vi "Upgraded_Live_Version.vi"() -> ()   [LabVIEW 2023]
panel:
  in  "Get ROI":bool
  in  "Height":u16
  in  "Y":u16
  in  "Width":u16
  in  "X":u16
  out "Trigger Mode":i32
  in  "Trigger In Behaviour":string(combo)
  out "Exp. out":i32
  in  "Trigger Out Behaviour":string(combo)
  out "Boolean":bool
  in  "Scan Direction Reset":bool
  out "Scan Line Time":dbl format="%#_14g"
  in  "Scan Width":dbl
  in  "Scan Line Delay":dbl
  in  "Scan Direction":string(combo)
  in  "Scan Mode":string(combo)
  in  "Exposure Time":dbl
  in  "Live":bool
  in  "Camera Status":bool
  in  "Uninit":bool
  in  "Live stop":bool
  in  "Live start":bool
  in  "Open":bool
  # "SimpleLiveAppProgrammableScanMode.vi\n\nDescription:\nThis sample code lets the user use programmable scan\n mode in an event driven structure.\n\nSteps to run:\n1. Click \"Run\"\n2. Click \"Open\"\n3. Enter Exposure Time\n4. Select Scan Mode. \n5. Set Scan Line Delay or Scan Width\n6. Select Scan Direction\n7. Click \"Live start\"\n8. Click \"Live stop\"\n9. Click \"Close\""
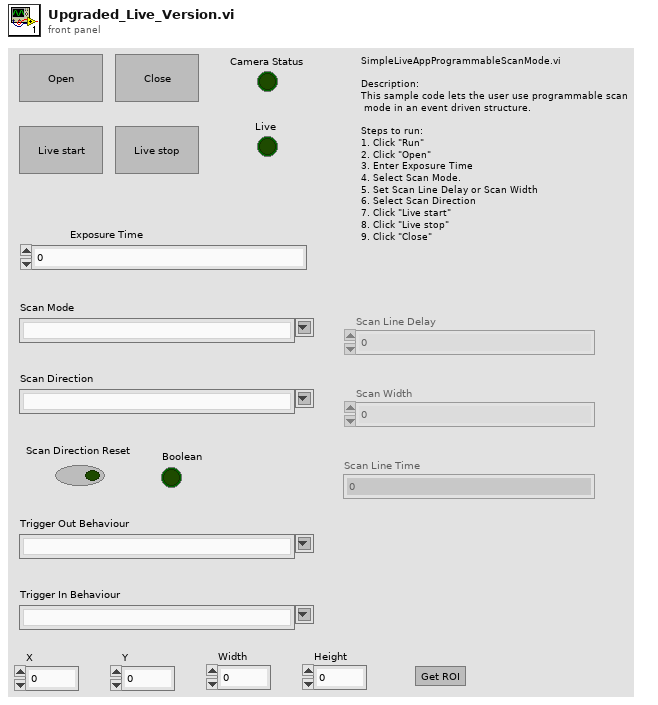
[diagram p1: front panel]
types:
  T1 = enum8{"Enabled", "Disabled", "Disabled and Grayed Out"}
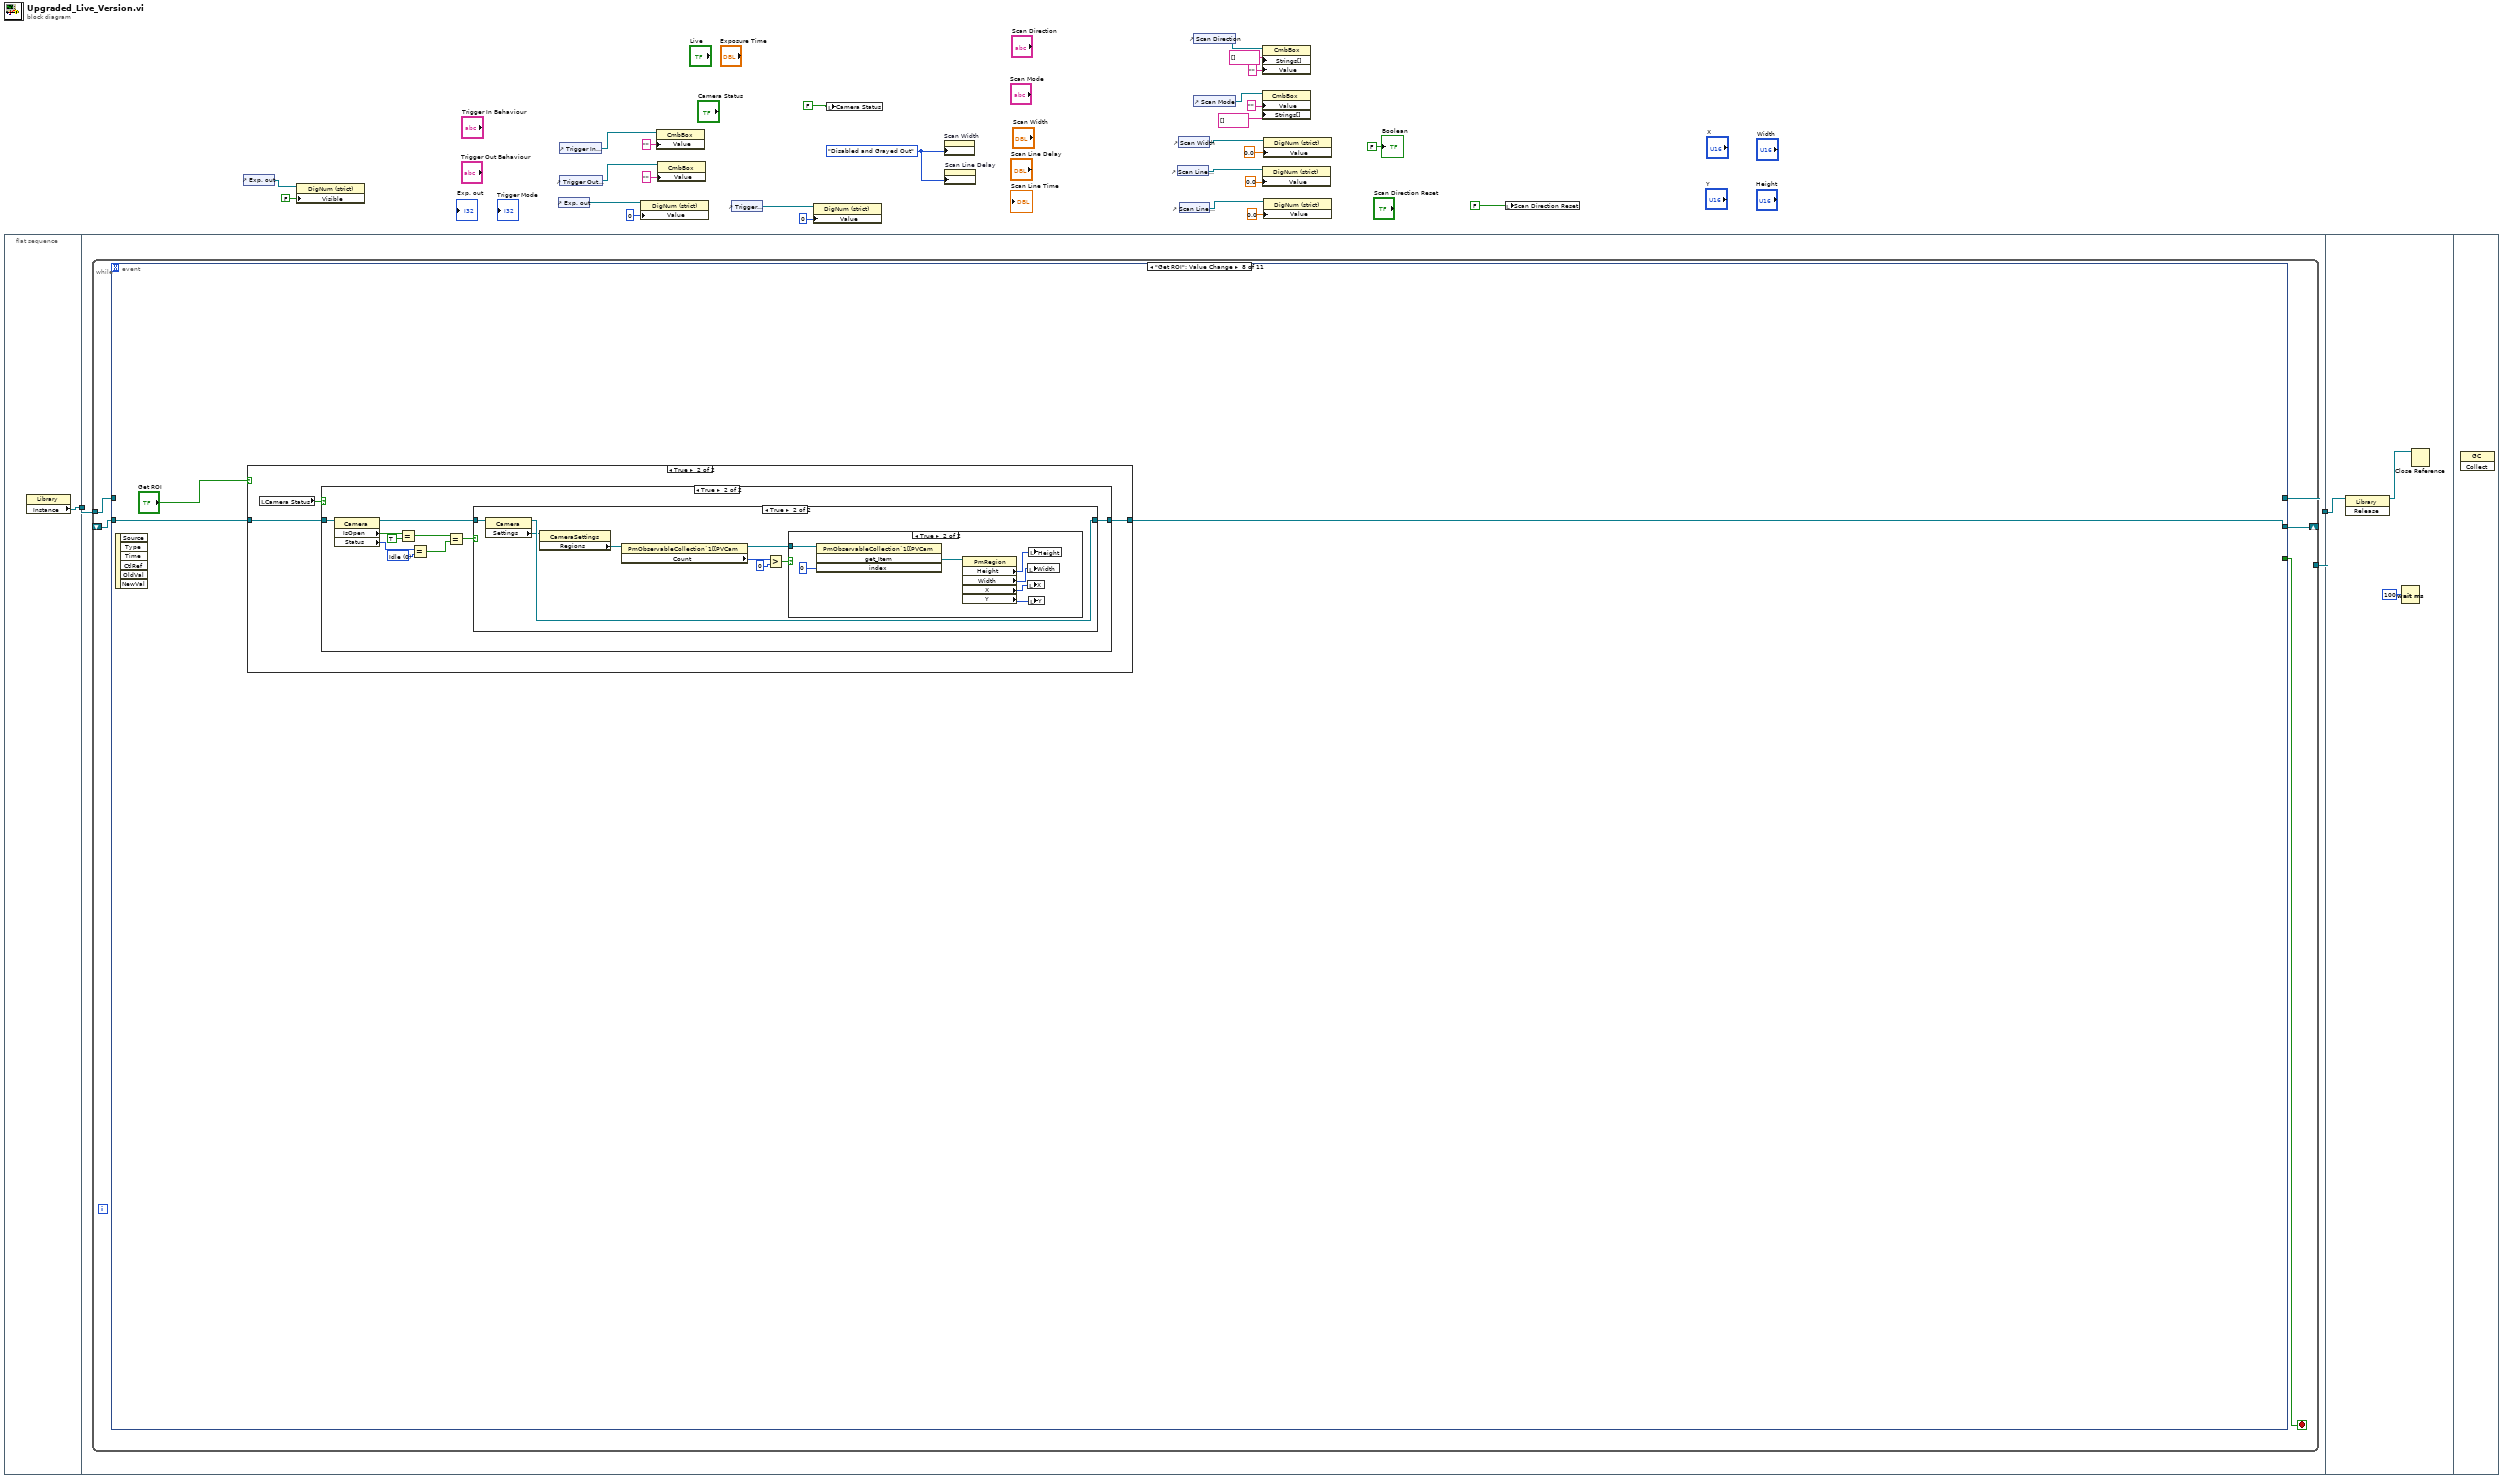
[diagram p0: block diagram]
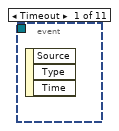
[diagram p2: hidden frame]
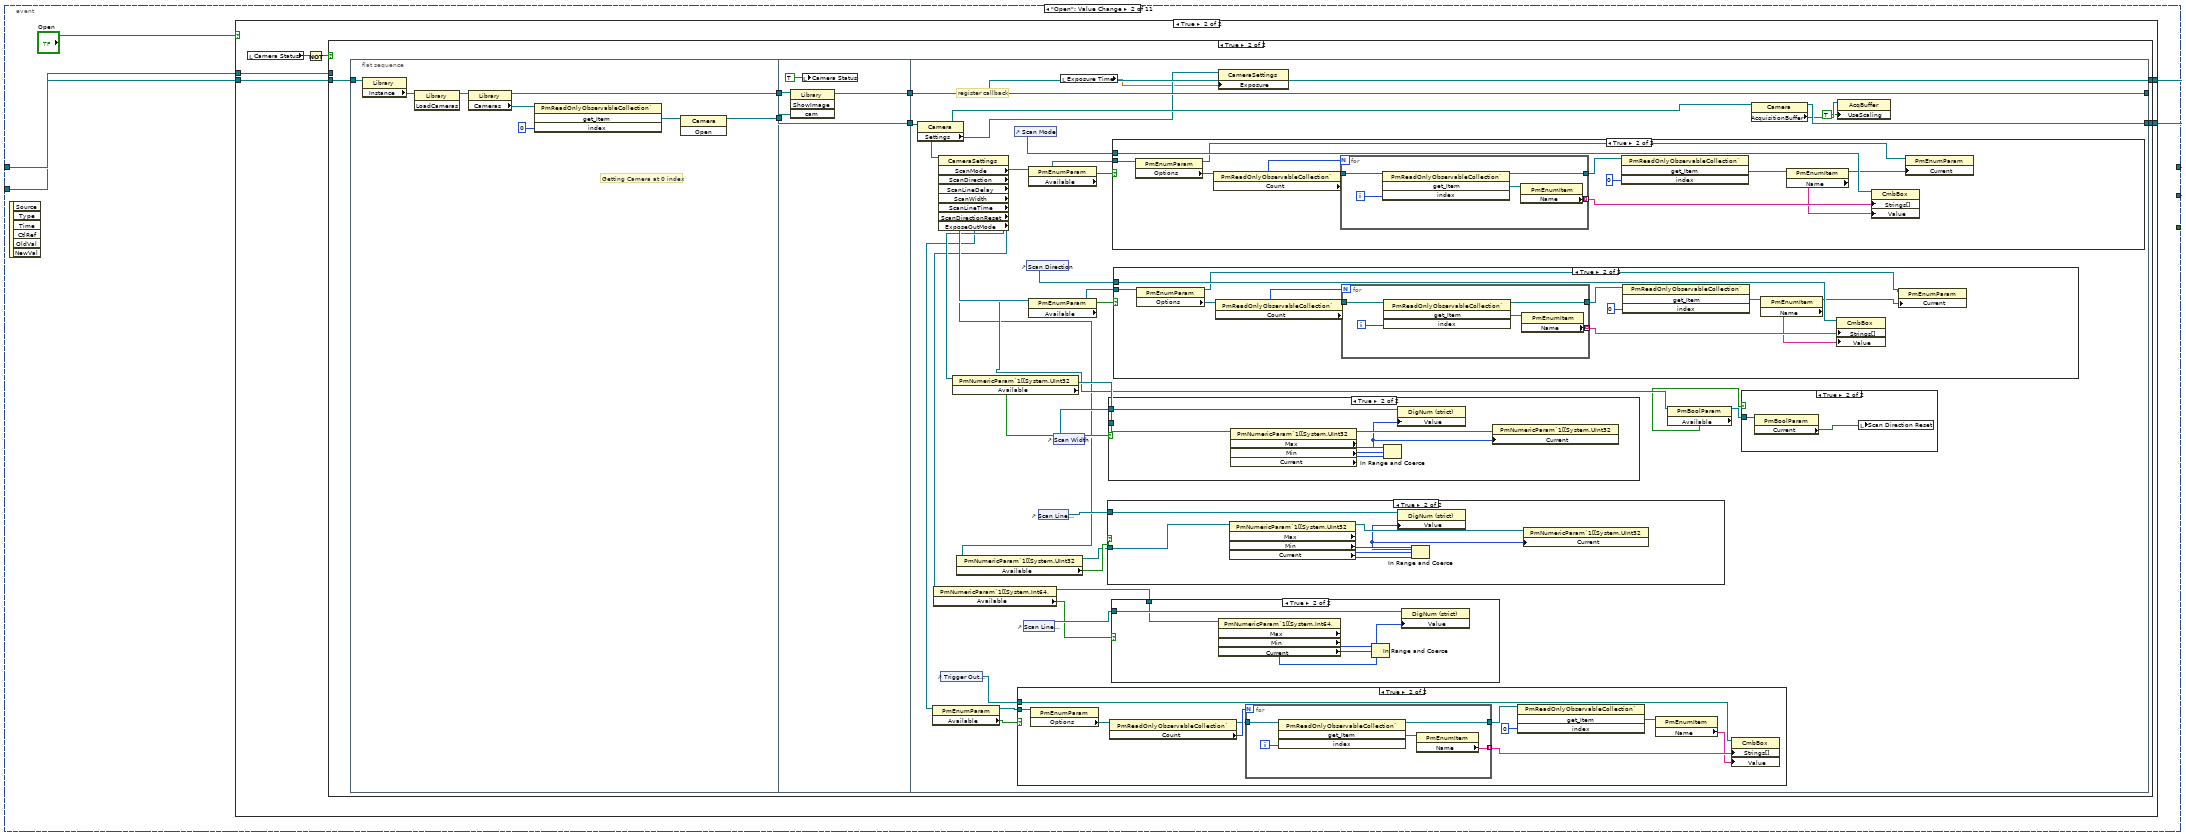
[diagram p3: hidden frame]
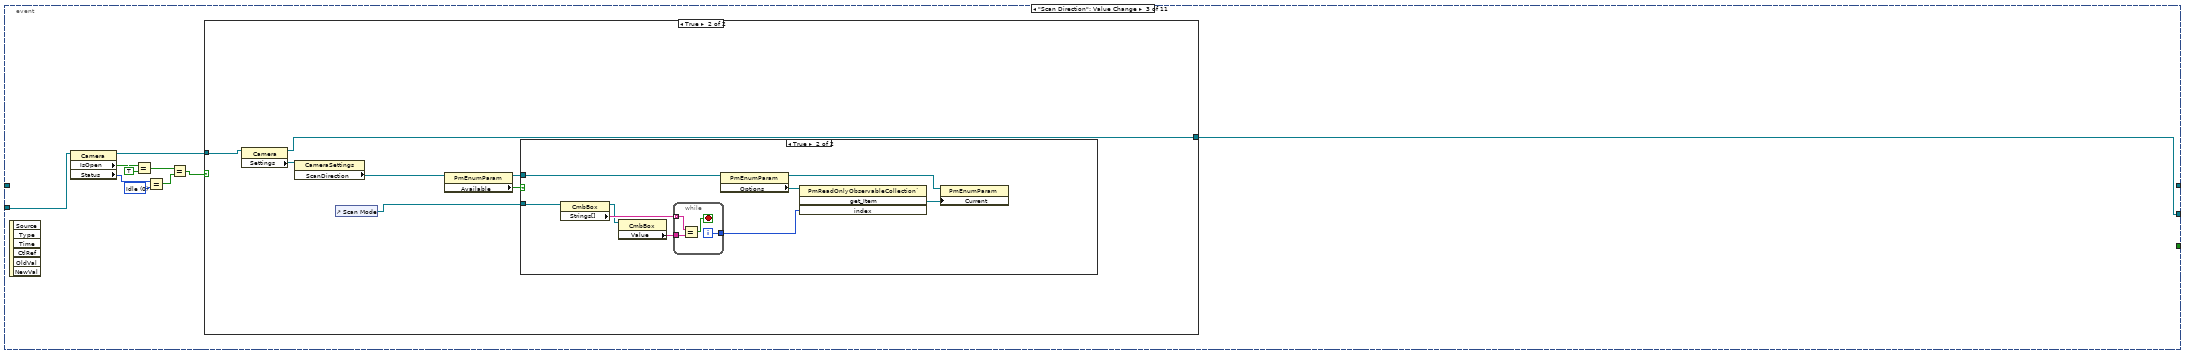
[diagram p13: hidden frame]
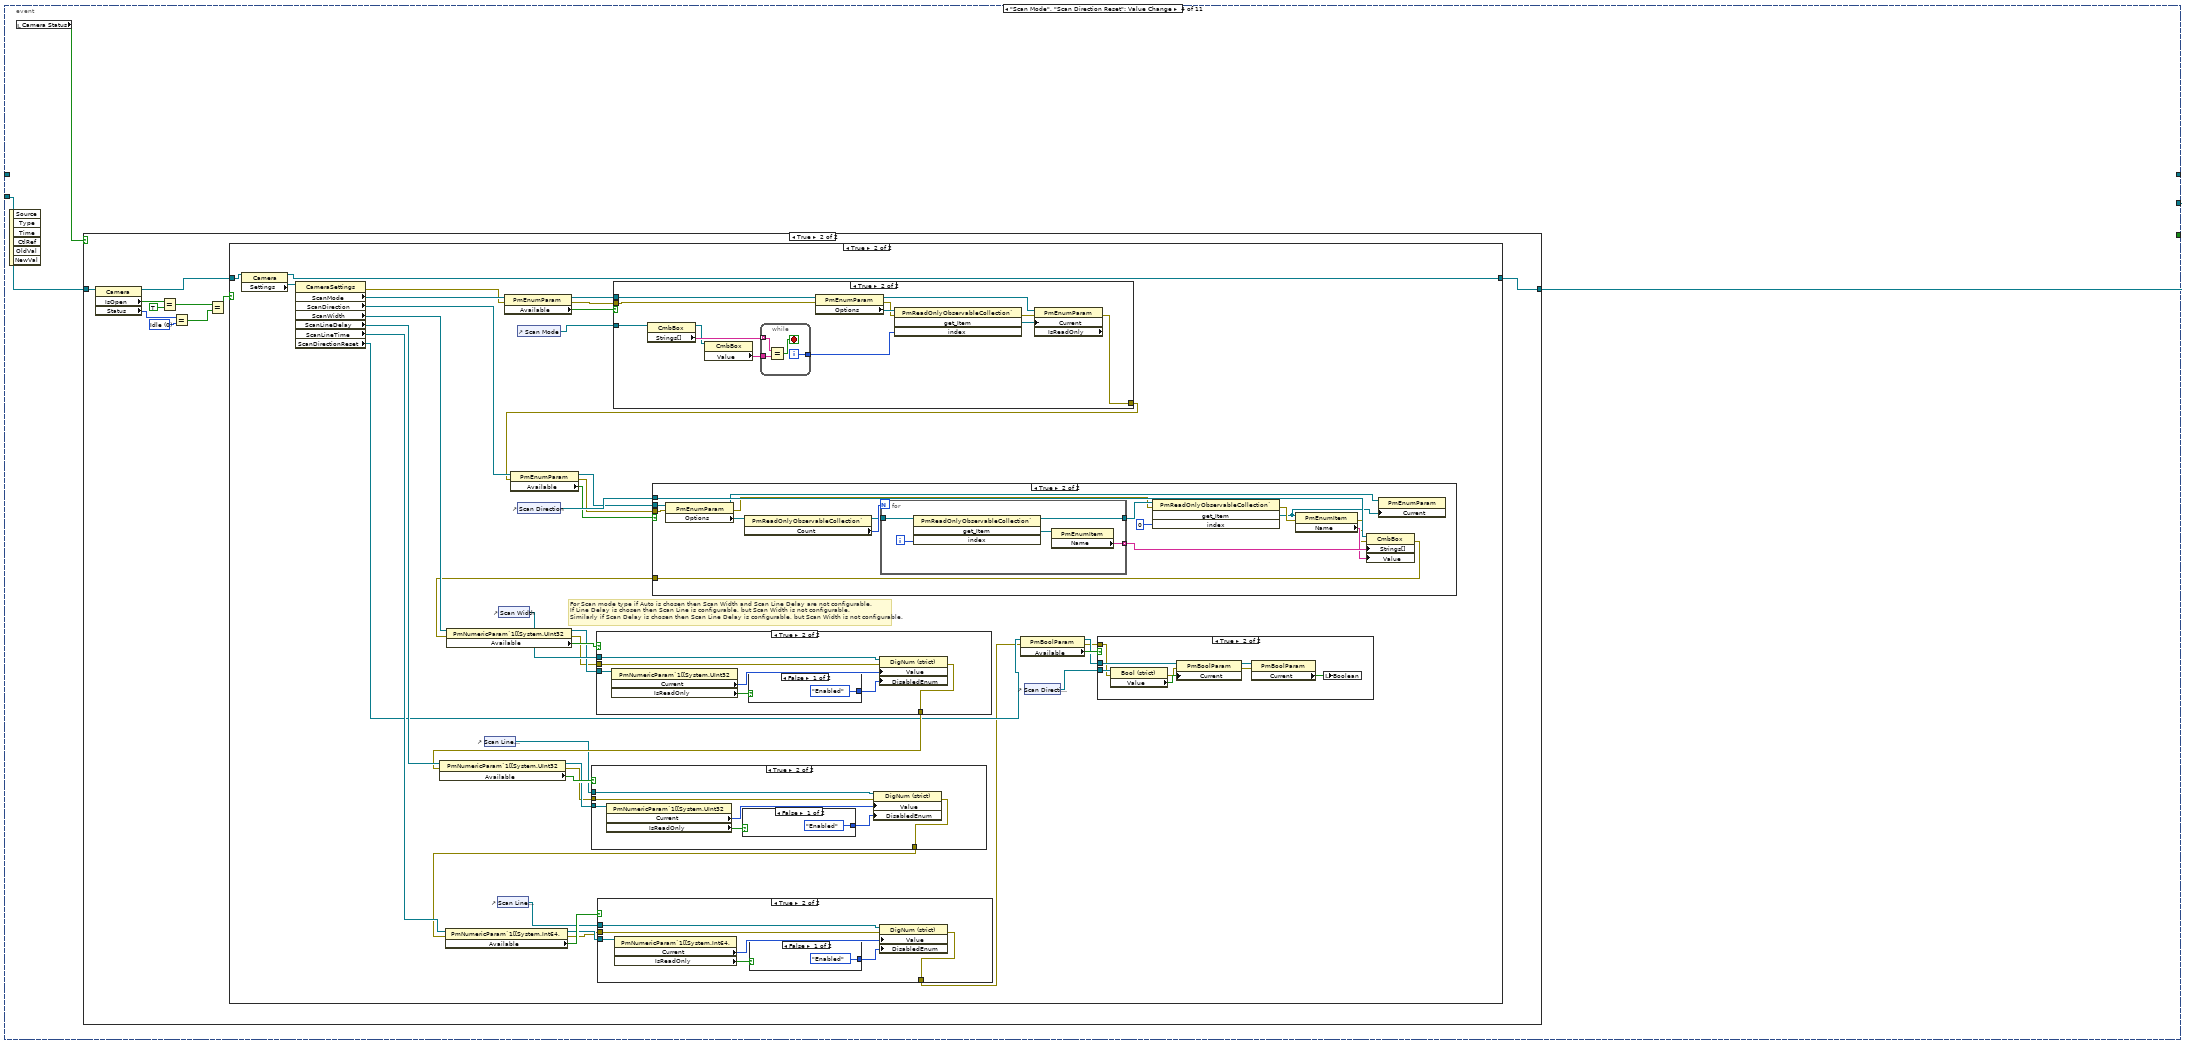
[diagram p16: hidden frame]
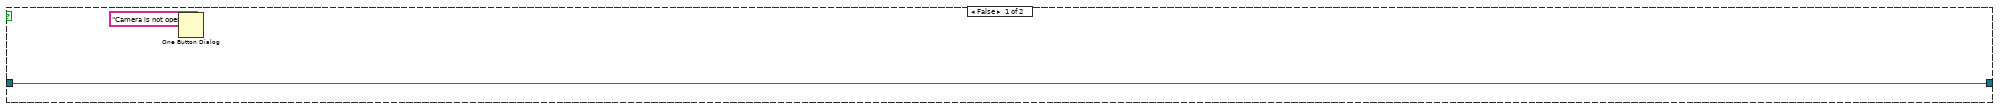
[diagram p17: hidden frame]
diagram:
  w13 = T1."Disabled and Grayed Out" ("Disabled")
  n1 = flat-sequence {
    tunnel: [w29] -> w28
    tunnel: w28 -> [w31]
    tunnel: [w30] -> w27
    tunnel: w27 -> [w652]
    frame #0 {
      n2 = property class="Library"() -> ("Instance"=w29:refnum<k24>)  [unwired: 2 in, 2 out]
    }
    frame #1 {
      n3 = while {
        tunnel: w31 -> [w36]
        shift-right: [w35] -> _
        shift-left: _ -> [w33]
        tunnel: [w34] -> w30
        stop <- w32 stop-if-true
        n4 = event shown="[7] \"Get ROI\": Value Change" {
          selector: _ -> [_ _ _ _ _ _ _ _ _ _ _]
          dyn-events: _ -> [_ _ _ _ _ _ _ _ _ _ _]
          timeout: _ -> [_ _ _ _ _ _ _ _ _ _ _]
          tunnel: w36 -> [_ w41 _ _ _ _ w464 _ w569 _ w624]
          tunnel: [_ w40 w177 w209 w341 w405 w465 w532 w570 w599 w625] -> w35
          tunnel: [_ w39 _ _ _ _ w464 _ w569 _ w624] -> w34
          tunnel: w33 -> [_ w38 w181 w210 w347 w407 w466 w533 w571 w600 w626]
          tunnel: [_ _ _ _ _ _ _ _ _ _ w623] -> w32
          event Timeout {
            n5 = event-data() -> ()  [unwired: 1 in, 3 out]
          }
          event "Open": Value Change {
            n6 = event-data() -> ()  [unwired: 1 in, 6 out]
            n7 = case shown="True" "Open" {
              tunnel: w41 -> [w43 w49]
              tunnel: [w42 w48] -> w40
              tunnel: [w43 w47] -> w39
              tunnel: w38 -> [w42 w44]
              frame False {
              }
              frame True {
                n8 = local read "Camera Status"() -> (w46:bool)
                n9 = Not(x=w46) -> (.not. x?=w45:bool)
                n10 = case shown="True" w45 {
                  tunnel: w49 -> [w50 w56]
                  tunnel: [w51 w55] -> w48
                  tunnel: [w50 w54] -> w47
                  tunnel: w44 -> [w51 _]
                  frame False {
                  }
                  frame True {
                    n11 = flat-sequence {
                      tunnel: w56 -> [w61]
                      tunnel: [w63] -> w58
                      tunnel: [w62] -> w57
                      tunnel: w58 -> [w69]
                      tunnel: w57 -> [w70]
                      tunnel: [w70] -> w53
                      tunnel: [w68] -> w52
                      tunnel: [w105] -> w54
                      tunnel: [w85] -> w55
                      tunnel: w53 -> [w104]
                      tunnel: w52 -> [w105]
                      frame #0 {
                        # "Getting Camera at 0 index"
                        n12 = property class="Library"(reference=w61) -> ("Instance"=w60:refnum<k24>)  [unwired: 1 in, 2 out]
                        n13 = invoke class="Library" method="LoadCameras"(reference=w60) -> (reference out=w59:refnum<k24>)  [unwired: 2 in, 2 out]
                        n14 = property class="Library"(reference=w59) -> (reference out=w63:refnum<k24>, "Cameras"=w66:refnum<k24>)  [unwired: 1 in, 1 out]
                        n15 = invoke class="PmReadOnlyObservableCollection`" method="get_Item"(reference=w66, "index"=0) -> ("get_Item"=w64:refnum<k24>)  [unwired: 2 in, 3 out]
                        n16 = invoke class="Camera" method="Open"(reference=w64) -> (reference out=w62:refnum<k24>)  [unwired: 2 in, 2 out]
                      }
                      frame #1 {
                        n17 = invoke class="Library" method="ShowImage"(reference=w69, "cam"=w70) -> (reference out=w68:refnum<k24>)  [unwired: 2 in, 3 out]
                        n18 = local write "Camera Status"(TRUE ("Camera Status")) -> ()
                      }
                      frame #2 {
                        # "register callback"
                        n19 = property class="Camera"(reference=w104) -> (reference out=w86:refnum<k24>, "Settings"=w75:refnum<k24>)  [unwired: 1 in, 1 out]
                        n20 = property class="CameraSettings"(reference=w75) -> ("ScanMode"=w103:refnum<k24>, "ScanDirection"=w99:refnum<k24>, "ScanLineDelay"=w94:refnum<k24>, "ScanWidth"=w81:refnum<k24>, "ScanLineTime"=w73:refnum<k24>, "ScanDirectionReset"=w89:refnum<k24>, "ExposeOutMode"=w77:refnum<k24>)  [unwired: 1 in, 2 out]
                        n21 = property class="PmEnumParam"(reference=w77) -> (reference out=w78:refnum<k24>, "Available"=w79:bool)  [unwired: 1 in, 1 out]
                        n22 = property class="PmNumericParam`1[[System.Int64,"(reference=w73) -> (reference out=w71:refnum<k24>, "Available"=w72:bool)  [unwired: 1 in, 1 out]
                        n23 = control-ref of="Trigger Out Behaviour"() -> (w76:refnum<vi>)
                        n24 = property class="PmNumericParam`1[[System.UInt32"(reference=w94) -> (reference out=w92:refnum<k24>, "Available"=w93:bool)  [unwired: 1 in, 1 out]
                        n25 = property class="PmNumericParam`1[[System.UInt32"(reference=w81) -> (reference out=w80:refnum<k24>, "Available"=w82:bool)  [unwired: 1 in, 1 out]
                        n26 = control-ref of="Scan Mode"() -> (w100:refnum<vi>)
                        n27 = case shown="True" w79 {
                          tunnel: w78 -> [_ w115]
                          tunnel: w76 -> [_ w106]
                          frame False {
                          }
                          frame True {
                            n28 = property class="PmEnumParam"(reference=w115) -> ("Options"=w114:refnum<k24>)  [unwired: 1 in, 2 out]
                            n29 = property class="PmReadOnlyObservableCollection`"(reference=w114) -> (reference out=w112:refnum<k24>, "Count"=w113:i32)  [unwired: 1 in, 1 out]
                            n30 = for {
                              N: w113 -> [_]
                              tunnel: w112 -> [w120]
                              tunnel: [w117] -> w109
                              tunnel: [w116] -> w108 mode=indexing
                              i -> [w119]
                              n31 = invoke class="PmReadOnlyObservableCollection`" method="get_Item"(reference=w120, "index"=w119) -> (reference out=w117:refnum<k24>, "get_Item"=w118:refnum<k24>)  [unwired: 2 in, 2 out]
                              n32 = property class="PmEnumItem"(reference=w118) -> ("Name"=w116:string)  [unwired: 1 in, 2 out]
                            }
                            n33 = invoke class="PmReadOnlyObservableCollection`" method="get_Item"(reference=w109, "index"=0) -> ("get_Item"=w110:refnum<k24>)  [unwired: 2 in, 3 out]
                            n34 = property class="PmEnumItem"(reference=w110) -> ("Name"=w107:string)  [unwired: 1 in, 2 out]
                            n35 = property class="CmbBox"(reference=w106, "Strings[]"=w108, "Value"=w107) -> ()  [unwired: 1 in, 2 out]
                          }
                        }
                        n36 = control-ref of="Scan Line Time"() -> (w90:refnum<vi>)
                        n37 = control-ref of="Scan Direction"() -> (w96:refnum<vi>)
                        n38 = property class="PmEnumParam"(reference=w103) -> (reference out=w101:refnum<k24>, "Available"=w102:bool)  [unwired: 1 in, 1 out]
                        n39 = property class="PmEnumParam"(reference=w99) -> (reference out=w97:refnum<k24>, "Available"=w98:bool)  [unwired: 1 in, 1 out]
                        n40 = control-ref of="Scan Line Delay"() -> (w91:refnum<vi>)
                        n41 = control-ref of="Scan Width"() -> (w95:refnum<vi>)
                        n42 = local read "Exposure Time"() -> (w74:dbl)
                        n43 = case shown="True" w82 {
                          tunnel: w91 -> [_ w132]
                          tunnel: w80 -> [_ w131]
                          frame False {
                          }
                          frame True {
                            n44 = property class="PmNumericParam`1[[System.UInt32"(reference=w131) -> (reference out=w130:refnum<k24>, "Max"=w133:u32, "Min"=w134:u32, "Current"=w135:u32)  [unwired: 1 in, 1 out]
                            n45 = In Range and Coerce(upper limit=w133, x=w135, lower limit=w134) -> (coerced(x)=w129:u32)  [unwired: 1 out]
                            n46 = property class="DigNum (strict)"(reference=w132, "Value"=w129) -> ()  [unwired: 1 in, 2 out]
                            n47 = property class="PmNumericParam`1[[System.UInt32"(reference=w130, "Current"=w129) -> ()  [unwired: 1 in, 2 out]
                          }
                        }
                        n48 = case shown="True" w93 {
                          tunnel: w95 -> [_ w139]
                          tunnel: w92 -> [_ w138]
                          frame False {
                          }
                          frame True {
                            n49 = property class="PmNumericParam`1[[System.UInt32"(reference=w138) -> (reference out=w137:refnum<k24>, "Max"=w140:u32, "Min"=w141:u32, "Current"=w142:u32)  [unwired: 1 in, 1 out]
                            n50 = In Range and Coerce(upper limit=w140, x=w142, lower limit=w141) -> (coerced(x)=w136:u32)  [unwired: 1 out]
                            n51 = property class="DigNum (strict)"(reference=w139, "Value"=w136) -> ()  [unwired: 1 in, 2 out]
                            n52 = property class="PmNumericParam`1[[System.UInt32"(reference=w137, "Current"=w136) -> ()  [unwired: 1 in, 2 out]
                          }
                        }
                        n53 = case shown="True" w72 {
                          tunnel: w90 -> [_ w124]
                          tunnel: w71 -> [_ w123]
                          frame False {
                          }
                          frame True {
                            n54 = property class="PmNumericParam`1[[System.Int64,"(reference=w123) -> ("Max"=w125:i64, "Min"=w126:i64, "Current"=w127:i64)  [unwired: 1 in, 2 out]
                            n55 = In Range and Coerce(upper limit=w125, x=w127, lower limit=w126) -> (coerced(x)=w128:i64)  [unwired: 1 out]
                            n56 = property class="DigNum (strict)"(reference=w124, "Value"=w128) -> ()  [unwired: 1 in, 2 out]
                          }
                        }
                        n57 = case shown="True" w102 {
                          tunnel: w101 -> [_ w171]
                          tunnel: w100 -> [_ w163]
                          frame False {
                          }
                          frame True {
                            n58 = property class="PmEnumParam"(reference=w171) -> (reference out=w162:refnum<k24>, "Options"=w170:refnum<k24>)  [unwired: 1 in, 1 out]
                            n59 = property class="PmReadOnlyObservableCollection`"(reference=w170) -> (reference out=w168:refnum<k24>, "Count"=w169:i32)  [unwired: 1 in, 1 out]
                            n60 = for {
                              N: w169 -> [_]
                              tunnel: w168 -> [w176]
                              tunnel: [w173] -> w166
                              tunnel: [w172] -> w165 mode=indexing
                              i -> [w175]
                              n61 = invoke class="PmReadOnlyObservableCollection`" method="get_Item"(reference=w176, "index"=w175) -> (reference out=w173:refnum<k24>, "get_Item"=w174:refnum<k24>)  [unwired: 2 in, 2 out]
                              n62 = property class="PmEnumItem"(reference=w174) -> ("Name"=w172:string)  [unwired: 1 in, 2 out]
                            }
                            n63 = invoke class="PmReadOnlyObservableCollection`" method="get_Item"(reference=w166, "index"=0) -> ("get_Item"=w161:refnum<k24>)  [unwired: 2 in, 3 out]
                            n64 = property class="PmEnumItem"(reference=w161) -> (reference out=w160:refnum<k24>, "Name"=w164:string)  [unwired: 1 in, 1 out]
                            n65 = property class="CmbBox"(reference=w163, "Strings[]"=w165, "Value"=w164) -> ()  [unwired: 1 in, 2 out]
                            n66 = property class="PmEnumParam"(reference=w162, "Current"=w160) -> ()  [unwired: 1 in, 2 out]
                          }
                        }
                        n67 = case shown="True" w98 {
                          tunnel: w97 -> [_ w154]
                          tunnel: w96 -> [_ w145]
                          frame False {
                          }
                          frame True {
                            n68 = property class="PmEnumParam"(reference=w154) -> (reference out=w144:refnum<k24>, "Options"=w153:refnum<k24>)  [unwired: 1 in, 1 out]
                            n69 = property class="PmReadOnlyObservableCollection`"(reference=w153) -> (reference out=w151:refnum<k24>, "Count"=w152:i32)  [unwired: 1 in, 1 out]
                            n70 = for {
                              N: w152 -> [_]
                              tunnel: w151 -> [w159]
                              tunnel: [w156] -> w148
                              tunnel: [w155] -> w147 mode=indexing
                              i -> [w158]
                              n71 = invoke class="PmReadOnlyObservableCollection`" method="get_Item"(reference=w159, "index"=w158) -> (reference out=w156:refnum<k24>, "get_Item"=w157:refnum<k24>)  [unwired: 2 in, 2 out]
                              n72 = property class="PmEnumItem"(reference=w157) -> ("Name"=w155:string)  [unwired: 1 in, 2 out]
                            }
                            n73 = invoke class="PmReadOnlyObservableCollection`" method="get_Item"(reference=w148, "index"=0) -> ("get_Item"=w149:refnum<k24>)  [unwired: 2 in, 3 out]
                            n74 = property class="PmEnumItem"(reference=w149) -> (reference out=w143:refnum<k24>, "Name"=w146:string)  [unwired: 1 in, 1 out]
                            n75 = property class="CmbBox"(reference=w145, "Strings[]"=w147, "Value"=w146) -> ()  [unwired: 1 in, 2 out]
                            n76 = property class="PmEnumParam"(reference=w144, "Current"=w143) -> ()  [unwired: 1 in, 2 out]
                          }
                        }
                        n77 = property class="CameraSettings"(reference=w75, "Exposure"=w74) -> ()  [unwired: 1 in, 2 out]
                        n78 = property class="PmBoolParam"(reference=w89) -> (reference out=w87:refnum<k24>, "Available"=w88:bool)  [unwired: 1 in, 1 out]
                        n79 = case shown="True" w88 {
                          tunnel: w87 -> [_ w122]
                          frame False {
                          }
                          frame True {
                            n80 = property class="PmBoolParam"(reference=w122) -> ("Current"=w121:bool)  [unwired: 1 in, 2 out]
                            n81 = local write "Scan Direction Reset"(w121) -> ()
                          }
                        }
                        n82 = property class="Camera"(reference=w86) -> (reference out=w85:refnum<k24>, "AcquisitionBuffer"=w84:refnum<k24>)  [unwired: 1 in, 1 out]
                        n83 = property class="AcqBuffer"(reference=w84, "UseScaling"=TRUE) -> ()  [unwired: 1 in, 2 out]
                      }
                    }
                  }
                }
              }
            }
          }
          event "Scan Direction": Value Change {
            w185 = 0 items=["Idle", "Capturing"] ("Status")
            n84 = event-data() -> ()  [unwired: 1 in, 6 out]
            n85 = property class="Camera"(reference=w181) -> (reference out=w178:refnum<k24>, "IsOpen"=w184:bool, "Status"=w186:i32)  [unwired: 1 in, 1 out]
            n86 = Equal?(x=w184, y=TRUE) -> (x = y?=w180:bool)
            n87 = Equal?(x=w186, y=w185) -> (x = y?=w182:bool)
            n88 = Equal?(x=w180, y=w182) -> (x = y?=w179:bool)
            n89 = case shown="True" w179 {
              tunnel: w178 -> [w187 w191]
              tunnel: [w187 w188] -> w177
              frame False {
              }
              frame True {
                n90 = property class="Camera"(reference=w191) -> (reference out=w188:refnum<k24>, "Settings"=w192:refnum<k24>)  [unwired: 1 in, 1 out]
                n91 = property class="CameraSettings"(reference=w192) -> ("ScanDirection"=w190:refnum<k24>)  [unwired: 1 in, 2 out]
                n92 = control-ref of="Scan Mode"() -> (w189:refnum<vi>)
                n93 = property class="PmEnumParam"(reference=w190) -> (reference out=w193:refnum<k24>, "Available"=w194:bool)  [unwired: 1 in, 1 out]
                n94 = case shown="True" w194 {
                  tunnel: w193 -> [_ w202]
                  tunnel: w189 -> [_ w195]
                  frame False {
                  }
                  frame True {
                    n95 = property class="CmbBox"(reference=w195) -> (reference out=w197:refnum<vi>, "Strings[]"=w203:string[])  [unwired: 1 in, 1 out]
                    n96 = property class="CmbBox"(reference=w197) -> ("Value"=w196:string)  [unwired: 1 in, 2 out]
                    n97 = while {
                      tunnel: w203 -> [w207] mode=indexing
                      tunnel: [w205] -> w200
                      tunnel: w196 -> [w204]
                      i -> [w205]
                      stop <- w206 stop-if-true
                      n98 = Equal?(x=w207, y=w204) -> (x = y?=w206:bool)
                    }
                    n99 = property class="PmEnumParam"(reference=w202) -> (reference out=w199:refnum<k24>, "Options"=w201:refnum<k24>)  [unwired: 1 in, 1 out]
                    n100 = invoke class="PmReadOnlyObservableCollection`" method="get_Item"(reference=w201, "index"=w200) -> ("get_Item"=w198:refnum<k24>)  [unwired: 2 in, 3 out]
                    n101 = property class="PmEnumParam"(reference=w199, "Current"=w198) -> ()  [unwired: 1 in, 2 out]
                  }
                }
              }
            }
          }
          event "Scan Mode", "Scan Direction Reset": Value Change {
            n102 = event-data() -> ()  [unwired: 1 in, 6 out]
            n103 = local read "Camera Status"() -> (w208:bool)
            n104 = case shown="True" w208 {
              tunnel: w210 -> [w211 w216]
              tunnel: [w211 w214] -> w209
              frame False {
                n105 = One Button Dialog(message="Camera is not open") -> ()  [unwired: 1 in, 1 out]
              }
              frame True {
                w221 = 0 items=["Idle", "Capturing"] ("Status")
                n106 = property class="Camera"(reference=w216) -> (reference out=w215:refnum<k24>, "IsOpen"=w220:bool, "Status"=w222:i32)  [unwired: 1 in, 1 out]
                n107 = Equal?(x=w220, y=TRUE) -> (x = y?=w218:bool)
                n108 = Equal?(x=w222, y=w221) -> (x = y?=w217:bool)
                n109 = Equal?(x=w218, y=w217) -> (x = y?=w213:bool)
                n110 = case shown="True" w213 {
                  tunnel: w215 -> [w223 w262]
                  tunnel: [w223 w257] -> w214
                  frame False {
                  }
                  frame True {
                    # "For Scan mode type if Auto is chosen then Scan Width and Scan Line Delay are not configurable.\nIf Line Delay is chosen then Scan Line is configurable, but Scan Width is not configurable.\nSimilarly if Scan Delay is chosen then Scan Line Delay is configurable, but Scan Width is not configurable."
                    n111 = property class="Camera"(reference=w262) -> (reference out=w257:refnum<k24>, "Settings"=w261:refnum<k24>)  [unwired: 1 in, 1 out]
                    n112 = property class="CameraSettings"(reference=w261) -> (error out=w254:errorcluster, "ScanMode"=w260:refnum<k24>, "ScanDirection"=w256:refnum<k24>, "ScanWidth"=w252:refnum<k24>, "ScanLineDelay"=w251:refnum<k24>, "ScanLineTime"=w240:refnum<k24>, "ScanDirectionReset"=w229:refnum<k24>)  [unwired: 1 in, 1 out]
                    n113 = control-ref of="Scan Line Delay"() -> (w231:refnum<vi>)
                    n114 = control-ref of="Scan Line Time"() -> (w234:refnum<vi>)
                    n115 = control-ref of="Scan Width"() -> (w247:refnum<vi>)
                    n116 = property class="PmEnumParam"(reference=w260, error in=w254) -> (reference out=w258:refnum<k24>, error out=w255:errorcluster, "Available"=w259:bool)
                    n117 = control-ref of="Scan Mode"() -> (w253:refnum<vi>)
                    n118 = control-ref of="Scan Direction"() -> (w250:refnum<vi>)
                    n119 = case shown="True" w259 {
                      tunnel: w258 -> [_ w335]
                      tunnel: w253 -> [_ w330]
                      tunnel: w255 -> [w323 w329]
                      tunnel: [w323 w324] -> w239
                      frame False {
                      }
                      frame True {
                        n120 = property class="CmbBox"(reference=w330) -> (reference out=w331:refnum<vi>, "Strings[]"=w336:string[])  [unwired: 1 in, 1 out]
                        n121 = property class="CmbBox"(reference=w331) -> ("Value"=w326:string)  [unwired: 1 in, 2 out]
                        n122 = while {
                          tunnel: w336 -> [w340] mode=indexing
                          tunnel: [w338] -> w333
                          tunnel: w326 -> [w337]
                          i -> [w338]
                          stop <- w339 stop-if-true
                          n123 = Equal?(x=w340, y=w337) -> (x = y?=w339:bool)
                        }
                        n124 = property class="PmEnumParam"(reference=w335, error in=w329) -> (reference out=w332:refnum<k24>, error out=w328:errorcluster, "Options"=w334:refnum<k24>)
                        n125 = invoke class="PmReadOnlyObservableCollection`" method="get_Item"(reference=w334, error in=w328, "index"=w333) -> (error out=w327:errorcluster, "get_Item"=w325:refnum<k24>)  [unwired: 1 in, 2 out]
                        n126 = property class="PmEnumParam" props=["Current", "IsReadOnly"](reference=w332, error in=w327, "Current"=w325) -> (error out=w324:errorcluster)  [unwired: 2 out]
                      }
                    }
                    n127 = property class="PmEnumParam"(reference=w256, error in=w239) -> (reference out=w248:refnum<k24>, error out=w242:errorcluster, "Available"=w249:bool)
                    n128 = case shown="True" w249 {
                      tunnel: w248 -> [_ w317]
                      tunnel: w250 -> [_ w309]
                      tunnel: w242 -> [w301 w308]
                      tunnel: [w301 w302] -> w241
                      frame False {
                      }
                      frame True {
                        n129 = property class="PmEnumParam"(reference=w317, error in=w308) -> (reference out=w303:refnum<k24>, error out=w307:errorcluster, "Options"=w316:refnum<k24>)
                        n130 = property class="PmReadOnlyObservableCollection`"(reference=w316) -> (reference out=w314:refnum<k24>, "Count"=w315:i32)  [unwired: 1 in, 1 out]
                        n131 = for {
                          N: w315 -> [_]
                          tunnel: w314 -> [w322]
                          tunnel: [w319] -> w312
                          tunnel: [w318] -> w311 mode=indexing
                          i -> [w321]
                          n132 = invoke class="PmReadOnlyObservableCollection`" method="get_Item"(reference=w322, "index"=w321) -> (reference out=w319:refnum<k24>, "get_Item"=w320:refnum<k24>)  [unwired: 2 in, 2 out]
                          n133 = property class="PmEnumItem"(reference=w320) -> ("Name"=w318:string)  [unwired: 1 in, 2 out]
                        }
                        n134 = invoke class="PmReadOnlyObservableCollection`" method="get_Item"(reference=w312, error in=w307, "index"=0) -> (error out=w306:errorcluster, "get_Item"=w304:refnum<k24>)  [unwired: 1 in, 2 out]
                        n135 = property class="PmEnumItem"(reference=w304, error in=w306) -> (error out=w305:errorcluster, "Name"=w310:string)  [unwired: 1 out]
                        n136 = property class="CmbBox"(reference=w309, error in=w305, "Strings[]"=w311, "Value"=w310) -> (error out=w302:errorcluster)  [unwired: 1 out]
                        n137 = property class="PmEnumParam"(reference=w303, "Current"=w304) -> ()  [unwired: 1 in, 2 out]
                      }
                    }
                    n138 = property class="PmNumericParam`1[[System.UInt32"(reference=w252, error in=w241) -> (reference out=w245:refnum<k24>, error out=w244:errorcluster, "Available"=w246:bool)
                    n139 = case shown="True" w246 {
                      tunnel: w247 -> [_ w297]
                      tunnel: w245 -> [_ w294]
                      tunnel: w244 -> [w291 w296]
                      tunnel: [w291 w295] -> w243
                      frame False {
                      }
                      frame True {
                        n140 = property class="PmNumericParam`1[[System.UInt32"(reference=w294) -> ("Current"=w298:u32, "IsReadOnly"=w293:bool)  [unwired: 1 in, 2 out]
                        n141 = case shown="False" w293 {
                          tunnel: [T1."Enabled" ("Disabled") T1."Disabled and Grayed Out" ("Disabled")] -> w292
                          frame False {
                          }
                          frame True {
                          }
                        }
                        n142 = property class="DigNum (strict)"(reference=w297, error in=w296, "Value"=w298, "DisabledEnum"=w292) -> (error out=w295:errorcluster)  [unwired: 1 out]
                      }
                    }
                    n143 = property class="PmNumericParam`1[[System.UInt32"(reference=w251, error in=w243) -> (reference out=w236:refnum<k24>, error out=w230:errorcluster, "Available"=w237:bool)
                    n144 = case shown="True" w237 {
                      tunnel: w231 -> [_ w287]
                      tunnel: w236 -> [_ w284]
                      tunnel: w230 -> [w281 w286]
                      tunnel: [w281 w285] -> w233
                      frame False {
                      }
                      frame True {
                        n145 = property class="PmNumericParam`1[[System.UInt32"(reference=w284) -> ("Current"=w288:u32, "IsReadOnly"=w283:bool)  [unwired: 1 in, 2 out]
                        n146 = case shown="False" w283 {
                          tunnel: [T1."Enabled" ("Disabled") T1."Disabled and Grayed Out" ("Disabled")] -> w282
                          frame False {
                          }
                          frame True {
                          }
                        }
                        n147 = property class="DigNum (strict)"(reference=w287, error in=w286, "Value"=w288, "DisabledEnum"=w282) -> (error out=w285:errorcluster)  [unwired: 1 out]
                      }
                    }
                    n148 = property class="PmNumericParam`1[[System.Int64,"(reference=w240, error in=w233) -> (reference out=w235:refnum<k24>, error out=w232:errorcluster, "Available"=w238:bool)
                    n149 = case shown="True" w238 {
                      tunnel: w234 -> [_ w277]
                      tunnel: w235 -> [_ w274]
                      tunnel: w232 -> [w271 w276]
                      tunnel: [w271 w275] -> w225
                      frame False {
                      }
                      frame True {
                        n150 = property class="PmNumericParam`1[[System.Int64,"(reference=w274) -> ("Current"=w278:i64, "IsReadOnly"=w273:bool)  [unwired: 1 in, 2 out]
                        n151 = case shown="False" w273 {
                          tunnel: [T1."Enabled" ("Disabled") T1."Disabled and Grayed Out" ("Disabled")] -> w272
                          frame False {
                          }
                          frame True {
                          }
                        }
                        n152 = property class="DigNum (strict)"(reference=w277, error in=w276, "Value"=w278, "DisabledEnum"=w272) -> (error out=w275:errorcluster)  [unwired: 1 out]
                      }
                    }
                    n153 = property class="PmBoolParam"(reference=w229, error in=w225) -> (reference out=w227:refnum<k24>, error out=w224:errorcluster, "Available"=w228:bool)
                    n154 = control-ref of="Scan Direction Reset"() -> (w226:refnum<vi>)
                    n155 = case shown="True" w228 {
                      tunnel: w227 -> [_ w268]
                      tunnel: w226 -> [_ w270]
                      tunnel: w224 -> [_ w265]
                      frame False {
                      }
                      frame True {
                        n156 = property class="Bool (strict)"(reference=w270, error in=w265) -> (error out=w264:errorcluster, "Value"=w269:bool)  [unwired: 1 out]
                        n157 = property class="PmBoolParam"(reference=w268, error in=w264, "Current"=w269) -> (reference out=w267:refnum<k24>, error out=w263:errorcluster)
                        n158 = property class="PmBoolParam"(reference=w267, error in=w263) -> ("Current"=w266:bool)  [unwired: 2 out]
                        n159 = local write "Boolean"(w266) -> ()
                      }
                    }
                  }
                }
              }
            }
          }
          event "Scan Line Delay": Value Change {
            w352 = 0 items=["Idle", "Capturing"] ("Status")
            n160 = event-data() -> ()  [unwired: 1 in, 6 out]
            n161 = property class="Camera"(reference=w347) -> (reference out=w346:refnum<k24>, "IsOpen"=w351:bool, "Status"=w353:i32)  [unwired: 1 in, 1 out]
            n162 = Equal?(x=w351, y=TRUE) -> (x = y?=w349:bool)
            n163 = Equal?(x=w353, y=w352) -> (x = y?=w348:bool)
            n164 = Equal?(x=w349, y=w348) -> (x = y?=w345:bool)
            n165 = control-ref of="Scan Line Time"() -> (w342:refnum<vi>)
            n166 = control-ref of="Scan Line Delay"() -> (w343:refnum<vi>)
            n167 = control-ref of="Scan Width"() -> (w344:refnum<vi>)
            n168 = case shown="True" w345 {
              tunnel: w346 -> [w354 w376]
              tunnel: [w354 w375] -> w341
              tunnel: w343 -> [_ w374]
              tunnel: w344 -> [_ w373]
              tunnel: w342 -> [_ w357]
              frame False {
              }
              frame True {
                n169 = property class="Camera"(reference=w376) -> (reference out=w375:refnum<k24>, "Settings"=w372:refnum<k24>)  [unwired: 1 in, 1 out]
                n170 = property class="CameraSettings"(reference=w372) -> (reference out=w362:refnum<k24>, error out=w368:errorcluster, "ScanLineDelay"=w371:refnum<k24>)  [unwired: 1 in]
                n171 = property class="PmNumericParam`1[[System.UInt32"(reference=w371, error in=w368) -> (reference out=w369:refnum<k24>, error out=w367:errorcluster, "Available"=w370:bool)
                n172 = case shown="True" w370 {
                  tunnel: w374 -> [_ w393]
                  tunnel: w369 -> [_ w392]
                  tunnel: w367 -> [w388 w391]
                  tunnel: [w388 w389] -> w363
                  frame False {
                  }
                  frame True {
                    n173 = property class="PmNumericParam`1[[System.UInt32"(reference=w392) -> (reference out=w396:refnum<k24>, "Max"=w394:u32, "Min"=w395:u32)  [unwired: 1 in, 1 out]
                    n174 = property class="DigNum (strict)"(reference=w393, error in=w391) -> (reference out=w400:refnum<vi>, error out=w390:errorcluster, "Value"=w399:dbl)
                    n175 = In Range and Coerce(upper limit=w394, x=w399, lower limit=w395) -> (coerced(x)=w398:dbl)  [unwired: 1 out]
                    n176 = property class="PmNumericParam`1[[System.UInt32"(reference=w396, "Current"=w398) -> (reference out=w397:refnum<k24>)  [unwired: 1 in, 1 out]
                    n177 = property class="PmNumericParam`1[[System.UInt32"(reference=w397) -> ("Current"=w401:u32)  [unwired: 1 in, 2 out]
                    n178 = property class="DigNum (strict)"(reference=w400, error in=w390, "Value"=w401) -> (error out=w389:errorcluster)  [unwired: 1 out]
                  }
                }
                n179 = property class="CameraSettings"(reference=w362) -> ("ScanWidth"=w361:refnum<k24>, "ScanLineTime"=w360:refnum<k24>)  [unwired: 1 in, 2 out]
                n180 = property class="PmNumericParam`1[[System.UInt32"(reference=w361, error in=w363) -> (reference out=w365:refnum<k24>, error out=w364:errorcluster, "Available"=w366:bool)
                n181 = case shown="True" w366 {
                  tunnel: w373 -> [_ w384]
                  tunnel: w365 -> [_ w387]
                  tunnel: w364 -> [w382 w385]
                  tunnel: [w382 w386] -> w356
                  frame False {
                  }
                  frame True {
                    n182 = property class="PmNumericParam`1[[System.UInt32"(reference=w387) -> ("Current"=w383:u32)  [unwired: 1 in, 2 out]
                    n183 = property class="DigNum (strict)"(reference=w384, error in=w385, "Value"=w383) -> (error out=w386:errorcluster)  [unwired: 1 out]
                  }
                }
                n184 = property class="PmNumericParam`1[[System.Int64,"(reference=w360, error in=w356) -> (reference out=w358:refnum<k24>, error out=w355:errorcluster, "Available"=w359:bool)
                n185 = case shown="True" w359 {
                  tunnel: w358 -> [_ w381]
                  tunnel: w357 -> [_ w379]
                  tunnel: w355 -> [_ w378]
                  frame False {
                  }
                  frame True {
                    n186 = property class="PmNumericParam`1[[System.Int64,"(reference=w381, error in=w378) -> (error out=w377:errorcluster, "Current"=w380:i64)  [unwired: 1 out]
                    n187 = property class="DigNum (strict)"(reference=w379, error in=w377, "Value"=w380) -> ()  [unwired: 2 out]
                  }
                }
              }
            }
          }
          event "Scan Width": Value Change {
            w413 = 0 items=["Idle", "Capturing"] ("Status")
            n188 = event-data() -> ()  [unwired: 1 in, 6 out]
            n189 = property class="Camera"(reference=w407) -> (reference out=w406:refnum<k24>, "IsOpen"=w412:bool, "Status"=w414:i32)  [unwired: 1 in, 1 out]
            n190 = Equal?(x=w412, y=TRUE) -> (x = y?=w410:bool)
            n191 = Equal?(x=w414, y=w413) -> (x = y?=w409:bool)
            n192 = Equal?(x=w410, y=w409) -> (x = y?=w408:bool)
            n193 = control-ref of="Scan Line Time"() -> (w402:refnum<vi>)
            n194 = control-ref of="Scan Width"() -> (w404:refnum<vi>)
            n195 = control-ref of="Scan Line Delay"() -> (w403:refnum<vi>)
            n196 = case shown="True" w408 {
              tunnel: w406 -> [w415 w437]
              tunnel: [w415 w436] -> w405
              tunnel: w404 -> [_ w435]
              tunnel: w403 -> [_ w434]
              tunnel: w402 -> [_ w419]
              frame False {
              }
              frame True {
                n197 = property class="Camera"(reference=w437) -> (reference out=w436:refnum<k24>, "Settings"=w433:refnum<k24>)  [unwired: 1 in, 1 out]
                n198 = property class="CameraSettings"(reference=w433) -> (reference out=w416:refnum<k24>, error out=w429:errorcluster, "ScanWidth"=w432:refnum<k24>)  [unwired: 1 in]
                n199 = property class="PmNumericParam`1[[System.UInt32"(reference=w432, error in=w429) -> (reference out=w430:refnum<k24>, error out=w428:errorcluster, "Available"=w431:bool)
                n200 = case shown="True" w431 {
                  tunnel: w435 -> [_ w454]
                  tunnel: w430 -> [_ w453]
                  tunnel: w428 -> [w449 w452]
                  tunnel: [w449 w450] -> w424
                  frame False {
                  }
                  frame True {
                    n201 = property class="PmNumericParam`1[[System.UInt32"(reference=w453) -> (reference out=w457:refnum<k24>, "Max"=w455:u32, "Min"=w456:u32)  [unwired: 1 in, 1 out]
                    n202 = property class="DigNum (strict)"(reference=w454, error in=w452) -> (reference out=w461:refnum<vi>, error out=w451:errorcluster, "Value"=w460:dbl)
                    n203 = In Range and Coerce(upper limit=w455, x=w460, lower limit=w456) -> (coerced(x)=w459:dbl)  [unwired: 1 out]
                    n204 = property class="PmNumericParam`1[[System.UInt32"(reference=w457, "Current"=w459) -> (reference out=w458:refnum<k24>)  [unwired: 1 in, 1 out]
                    n205 = property class="PmNumericParam`1[[System.UInt32"(reference=w458) -> ("Current"=w462:u32)  [unwired: 1 in, 2 out]
                    n206 = property class="DigNum (strict)"(reference=w461, error in=w451, "Value"=w462) -> (error out=w450:errorcluster)  [unwired: 1 out]
                  }
                }
                n207 = property class="CameraSettings"(reference=w416) -> ("ScanLineDelay"=w423:refnum<k24>, "ScanLineTime"=w422:refnum<k24>)  [unwired: 1 in, 2 out]
                n208 = property class="PmNumericParam`1[[System.UInt32"(reference=w423, error in=w424) -> (reference out=w426:refnum<k24>, error out=w425:errorcluster, "Available"=w427:bool)
                n209 = case shown="True" w427 {
                  tunnel: w434 -> [_ w445]
                  tunnel: w426 -> [_ w448]
                  tunnel: w425 -> [w443 w446]
                  tunnel: [w443 w447] -> w418
                  frame False {
                  }
                  frame True {
                    n210 = property class="PmNumericParam`1[[System.UInt32"(reference=w448) -> ("Current"=w444:u32)  [unwired: 1 in, 2 out]
                    n211 = property class="DigNum (strict)"(reference=w445, error in=w446, "Value"=w444) -> (error out=w447:errorcluster)  [unwired: 1 out]
                  }
                }
                n212 = property class="PmNumericParam`1[[System.Int64,"(reference=w422, error in=w418) -> (reference out=w420:refnum<k24>, error out=w417:errorcluster, "Available"=w421:bool)
                n213 = case shown="True" w421 {
                  tunnel: w420 -> [_ w442]
                  tunnel: w419 -> [_ w440]
                  tunnel: w417 -> [_ w439]
                  frame False {
                  }
                  frame True {
                    n214 = property class="PmNumericParam`1[[System.Int64,"(reference=w442, error in=w439) -> (error out=w438:errorcluster, "Current"=w441:i64)  [unwired: 1 out]
                    n215 = property class="DigNum (strict)"(reference=w440, error in=w438, "Value"=w441) -> ()  [unwired: 2 out]
                  }
                }
              }
            }
          }
          event "Exposure Time", "Trigger Out Behaviour", "Trigger In Behaviour": Value Change {
            n216 = event-data() -> ()  [unwired: 1 in, 6 out]
            n217 = local read "Camera Status"() -> (w463:bool)
            n218 = case shown="True" w463 {
              tunnel: w466 -> [w468 w472]
              tunnel: [w468 w469] -> w465
              frame False {
                n219 = One Button Dialog(message="Camera is not open") -> ()  [unwired: 1 in, 1 out]
              }
              frame True {
                w477 = 0 items=["Idle", "Capturing"] ("Status")
                n220 = property class="Camera"(reference=w472) -> (reference out=w470:refnum<k24>, "IsOpen"=w476:bool, "Status"=w478:i32)  [unwired: 1 in, 1 out]
                n221 = Equal?(x=w476, y=TRUE) -> (x = y?=w474:bool)
                n222 = Equal?(x=w478, y=w477) -> (x = y?=w473:bool)
                n223 = Equal?(x=w474, y=w473) -> (x = y?=w471:bool)
                n224 = case shown="True" w471 {
                  tunnel: w470 -> [w479 w501]
                  tunnel: [w479 w493] -> w469
                  frame False {
                  }
                  frame True {
                    n225 = property class="Camera"(reference=w501) -> (reference out=w493:refnum<k24>, "Settings"=w488:refnum<k24>)  [unwired: 1 in, 1 out]
                    n226 = control-ref of="Trigger Mode"() -> (w483:refnum<vi>)
                    n227 = control-ref of="Trigger In Behaviour"() -> (w482:refnum<vi>)
                    n228 = control-ref of="Exp. out"() -> (w490:refnum<vi>)
                    n229 = control-ref of="Trigger Out Behaviour"() -> (w489:refnum<vi>)
                    n230 = property class="CameraSettings"(reference=w488) -> (reference out=w487:refnum<k24>, "ExposureTime"=w486:refnum<k24>, "ExposureMode"=w480:refnum<k24>, "ExposeOutMode"=w485:refnum<k24>)  [unwired: 1 in, 1 out]
                    n231 = property class="PmEnumParam"(reference=w480) -> (reference out=w484:refnum<k24>, "Available"=w481:bool)  [unwired: 1 in, 1 out]
                    n232 = property class="PmEnumParam"(reference=w485) -> (reference out=w491:refnum<k24>, "Available"=w492:bool)  [unwired: 1 in, 1 out]
                    n233 = property class="PmNumericParam`1[[System.UInt64"(reference=w486) -> (reference out=w498:refnum<k24>, "Max"=w500:u64, "Min"=w499:u64)  [unwired: 1 in, 1 out]
                    n234 = case shown="True" w492 {
                      tunnel: w491 -> [_ w526]
                      tunnel: w490 -> [_ w520]
                      tunnel: w489 -> [_ w517]
                      frame False {
                      }
                      frame True {
                        n235 = property class="CmbBox"(reference=w517) -> (reference out=w519:refnum<vi>, "Strings[]"=w527:string[])  [unwired: 1 in, 1 out]
                        n236 = property class="CmbBox"(reference=w519) -> ("Value"=w518:string)  [unwired: 1 in, 2 out]
                        n237 = while {
                          tunnel: w527 -> [w531] mode=indexing
                          tunnel: [w529] -> w524
                          tunnel: w518 -> [w528]
                          i -> [w529]
                          stop <- w530 stop-if-true
                          n238 = Equal?(x=w531, y=w528) -> (x = y?=w530:bool)
                        }
                        n239 = property class="PmEnumParam"(reference=w526) -> (reference out=w523:refnum<k24>, "Options"=w525:refnum<k24>)  [unwired: 1 in, 1 out]
                        n240 = invoke class="PmReadOnlyObservableCollection`" method="get_Item"(reference=w525, "index"=w524) -> ("get_Item"=w522:refnum<k24>)  [unwired: 2 in, 3 out]
                        n241 = property class="PmEnumItem"(reference=w522) -> ("Value"=w521:i32)  [unwired: 1 in, 2 out]
                        n242 = property class="PmEnumParam"(reference=w523, "Current"=w522) -> ()  [unwired: 1 in, 2 out]
                        n243 = property class="DigNum (strict)"(reference=w520, "Value"=w521) -> ()  [unwired: 1 in, 2 out]
                      }
                    }
                    n244 = case shown="True" w481 {
                      tunnel: w483 -> [_ w506]
                      tunnel: w482 -> [_ w503]
                      tunnel: w484 -> [_ w502]
                      frame False {
                      }
                      frame True {
                        n245 = property class="CmbBox"(reference=w503) -> (reference out=w505:refnum<vi>, "Strings[]"=w512:string[])  [unwired: 1 in, 1 out]
                        n246 = property class="CmbBox"(reference=w505) -> ("Value"=w504:string)  [unwired: 1 in, 2 out]
                        n247 = while {
                          tunnel: w512 -> [w516] mode=indexing
                          tunnel: [w514] -> w510
                          tunnel: w504 -> [w513]
                          i -> [w514]
                          stop <- w515 stop-if-true
                          n248 = Equal?(x=w516, y=w513) -> (x = y?=w515:bool)
                        }
                        n249 = property class="PmEnumParam"(reference=w502) -> (reference out=w509:refnum<k24>, "Options"=w511:refnum<k24>)  [unwired: 1 in, 1 out]
                        n250 = invoke class="PmReadOnlyObservableCollection`" method="get_Item"(reference=w511, "index"=w510) -> ("get_Item"=w508:refnum<k24>)  [unwired: 2 in, 3 out]
                        n251 = property class="PmEnumItem"(reference=w508) -> ("Value"=w507:i32)  [unwired: 1 in, 2 out]
                        n252 = property class="PmEnumParam"(reference=w509, "Current"=w508) -> ()  [unwired: 1 in, 2 out]
                        n253 = property class="DigNum (strict)"(reference=w506, "Value"=w507) -> ()  [unwired: 1 in, 2 out]
                      }
                    }
                    n254 = local read "Exposure Time"() -> (w495:dbl)
                    n255 = In Range and Coerce(upper limit=w500, x=w495, lower limit=w499) -> (coerced(x)=w496:dbl)  [unwired: 1 out]
                    n256 = property class="CameraSettings"(reference=w487, "Exposure"=w496) -> ()  [unwired: 1 in, 2 out]
                    n257 = property class="PmNumericParam`1[[System.UInt64"(reference=w498, "Current"=w496) -> (reference out=w497:refnum<k24>)  [unwired: 1 in, 1 out]
                    n258 = property class="PmNumericParam`1[[System.UInt64"(reference=w497) -> ("Current"=w494:u64)  [unwired: 1 in, 2 out]
                    n259 = local write "Exposure Time"(w494) -> ()
                  }
                }
              }
            }
          }
          event "Get ROI": Value Change {
            n260 = event-data() -> ()  [unwired: 1 in, 6 out]
            n261 = case shown="True" "Get ROI" {
              tunnel: w533 -> [w535 w538]
              tunnel: [w535 w537] -> w532
              frame False {
              }
              frame True {
                n262 = local read "Camera Status"() -> (w536:bool)
                n263 = case shown="True" w536 {
                  tunnel: w538 -> [w540 w544]
                  tunnel: [w540 w541] -> w537
                  frame False {
                    n264 = One Button Dialog(message="Camera is not open") -> ()  [unwired: 1 in, 1 out]
                  }
                  frame True {
                    w549 = 0 items=["Idle", "Capturing"] ("Status")
                    n265 = property class="Camera"(reference=w544) -> (reference out=w543:refnum<k24>, "IsOpen"=w548:bool, "Status"=w550:i32)  [unwired: 1 in, 1 out]
                    n266 = Equal?(x=w548, y=TRUE) -> (x = y?=w546:bool)
                    n267 = Equal?(x=w550, y=w549) -> (x = y?=w545:bool)
                    n268 = Equal?(x=w546, y=w545) -> (x = y?=w542:bool)
                    n269 = case shown="True" w542 {
                      tunnel: w543 -> [w552 w560]
                      tunnel: [w552 w559] -> w541
                      frame False {
                        n270 = One Button Dialog(message="Camera must be idle.") -> ()  [unwired: 1 in, 1 out]
                      }
                      frame True {
                        n271 = property class="Camera"(reference=w560) -> (reference out=w559:refnum<k24>, "Settings"=w558:refnum<k24>)  [unwired: 1 in, 1 out]
                        n272 = property class="CameraSettings"(reference=w558) -> ("Regions"=w557:refnum<k24>)  [unwired: 1 in, 2 out]
                        n273 = property class="PmObservableCollection`1[[PVCam"(reference=w557) -> (reference out=w553:refnum<k24>, "Count"=w556:i32)  [unwired: 1 in, 1 out]
                        n274 = Greater?(x=w556, y=0) -> (0:w554:bool)
                        n275 = case shown="True" w554 {
                          tunnel: w553 -> [_ w562]
                          frame False {
                            n276 = One Button Dialog(message="ROI is not created.") -> ()  [unwired: 1 in, 1 out]
                          }
                          frame True {
                            n277 = invoke class="PmObservableCollection`1[[PVCam" method="get_Item"(reference=w562, "index"=0) -> ("get_Item"=w568:refnum<k24>)  [unwired: 2 in, 3 out]
                            n278 = property class="PmRegion"(reference=w568) -> ("Height"=w566:u16, "Width"=w565:u16, "X"=w564:u16, "Y"=w563:u16)  [unwired: 1 in, 2 out]
                            n279 = local write "Width"(w565) -> ()
                            n280 = local write "X"(w564) -> ()
                            n281 = local write "Height"(w566) -> ()
                            n282 = local write "Y"(w563) -> ()
                          }
                        }
                      }
                    }
                  }
                }
              }
            }
          }
          event "Live start": Value Change {
            n283 = event-data() -> ()  [unwired: 1 in, 6 out]
            n284 = case shown="True" "Live start" {
              tunnel: w571 -> [w573 w576]
              tunnel: [w573 w575] -> w570
              frame False {
              }
              frame True {
                n285 = local read "Camera Status"() -> (w574:bool)
                n286 = case shown="True" w574 {
                  tunnel: w576 -> [w577 w582]
                  tunnel: [w577 w580] -> w575
                  frame False {
                    n287 = One Button Dialog(message="Camera is not open") -> ()  [unwired: 1 in, 1 out]
                  }
                  frame True {
                    w587 = 0 items=["Idle", "Capturing"] ("Status")
                    n288 = property class="Camera"(reference=w582) -> (reference out=w581:refnum<k24>, "IsOpen"=w586:bool, "Status"=w588:i32)  [unwired: 1 in, 1 out]
                    n289 = Equal?(x=w586, y=TRUE) -> (x = y?=w584:bool)
                    n290 = Equal?(x=w588, y=w587) -> (x = y?=w583:bool)
                    n291 = Equal?(x=w584, y=w583) -> (x = y?=w579:bool)
                    n292 = case shown="True" w579 {
                      tunnel: w581 -> [w590 w592]
                      tunnel: [w590 w593] -> w580
                      frame False {
                        n293 = local write "Live"(FALSE ("Live 2")) -> ()
                      }
                      frame True {
                        n294 = flat-sequence {
                          tunnel: w592 -> [w598]
                          tunnel: [w595] -> w591
                          frame #0 {
                            n295 = property class="Camera"(reference=w598) -> (reference out=w595:refnum<k24>, "AcquisitionBuffer"=w597:refnum<k24>)  [unwired: 1 in, 1 out]
                            n296 = property class="AcqBuffer"(reference=w597, "BufferSize"=100) -> ()  [unwired: 1 in, 2 out]
                          }
                        }
                        n297 = local write "Live"(TRUE ("Live")) -> ()
                        n298 = invoke class="Camera" method="StartLive"(reference=w591) -> (reference out=w593:refnum<k24>)  [unwired: 2 in, 2 out]
                      }
                    }
                  }
                }
              }
            }
          }
          event "Live stop": Value Change {
            n299 = event-data() -> ()  [unwired: 1 in, 6 out]
            n300 = case shown="True" "Live stop" {
              tunnel: w600 -> [w602 w605]
              tunnel: [w602 w604] -> w599
              frame False {
              }
              frame True {
                n301 = local read "Camera Status"() -> (w603:bool)
                n302 = case shown="False" w603 {
                  tunnel: w605 -> [w607 w617]
                  tunnel: [w607 w614] -> w604
                  frame False {
                    n303 = One Button Dialog(message="Camera is not open") -> ()  [unwired: 1 in, 1 out]
                  }
                  frame True {
                    w612 = 1 items=["Idle", "Capturing"] ("Status")
                    n304 = property class="Camera"(reference=w617) -> (reference out=w615:refnum<k24>, "IsOpen"=w611:bool, "Status"=w613:i32)  [unwired: 1 in, 1 out]
                    n305 = Equal?(x=w613, y=w612) -> (x = y?=w608:bool)
                    n306 = Equal?(x=w611, y=TRUE) -> (x = y?=w609:bool)
                    n307 = Equal?(x=w609, y=w608) -> (x = y?=w616:bool)
                    n308 = case shown="True" w616 {
                      tunnel: w615 -> [w618 w621]
                      tunnel: [w618 w620] -> w614
                      frame False {
                      }
                      frame True {
                        n309 = invoke class="Camera" method="Stop"(reference=w621) -> (reference out=w620:refnum<k24>)  [unwired: 2 in, 2 out]
                        n310 = local write "Live"(FALSE ("Live 2")) -> ()
                      }
                    }
                  }
                }
              }
            }
          }
          event "Uninit": Value Change {
            n311 = event-data() -> ()  [unwired: 1 in, 6 out]
            n312 = case shown="True" "Uninit" {
              tunnel: w626 -> [w628 w632]
              tunnel: [w628 w631] -> w625
              tunnel: [FALSE ("Camera Status") w629] -> w623
              frame False {
              }
              frame True {
                n313 = local read "Camera Status"() -> (w630:bool)
                n314 = case shown="True" w630 {
                  tunnel: w632 -> [w634 w639]
                  tunnel: [w634 w638] -> w631
                  tunnel: [FALSE ("Camera Status") w637] -> w629
                  frame False {
                  }
                  frame True {
                    n315 = local read "Live"() -> (w635:bool)
                    n316 = Not(x=w635) -> (.not. x?=w636:bool)
                    n317 = case shown="True" w636 {
                      tunnel: w639 -> [w641 w644]
                      tunnel: [w641 w643] -> w638
                      tunnel: [FALSE ("Camera Status") w642] -> w637
                      frame False {
                      }
                      frame True {
                        n318 = flat-sequence {
                          tunnel: w644 -> [w647]
                          tunnel: [w646] -> w645
                          tunnel: [w650] -> w643
                          tunnel: w645 -> [w650]
                          tunnel: [TRUE ("Camera Status")] -> w642
                          frame #0 {
                            n319 = invoke class="Camera" method="Close"(reference=w647) -> (reference out=w646:refnum<k24>)  [unwired: 2 in, 2 out]
                          }
                          frame #1 {
                            n320 = local write "Camera Status"(FALSE ("Camera Status")) -> ()
                          }
                        }
                      }
                    }
                  }
                }
              }
            }
          }
        }
      }
    }
    frame #2 {
      n321 = invoke class="Library" method="Release"(reference=w652) -> (reference out=w653:refnum<k24>)  [unwired: 2 in, 2 out]
      n322 = Wait (ms)(milliseconds to wait=u32 100) -> ()  [unwired: 1 out]
      n323 = Close Reference(reference=w653) -> ()  [unwired: 1 in, 1 out]
    }
    frame #3 {
      n324 = invoke class="GC" method="Collect"() -> ()  [unwired: 3 in, 3 out]
    }
  }
  n325 = control-ref of="Exp. out"() -> (w5:refnum<vi>)
  n326 = property class="DigNum (strict)"(reference=w5, "Visible"=FALSE) -> ()  [unwired: 1 in, 2 out]
  n327 = control-ref of="Exp. out"() -> (w8:refnum<vi>)
  n328 = control-ref of="Trigger In Behaviour"() -> (w4:refnum<vi>)
  n329 = control-ref of="Trigger Out Behaviour"() -> (w10:refnum<vi>)
  n330 = property class="DigNum (strict)"(reference=w8, "Value"=0) -> ()  [unwired: 1 in, 2 out]
  n331 = property class="CmbBox"(reference=w4, "Value"="") -> ()  [unwired: 1 in, 2 out]
  n332 = property class="CmbBox"(reference=w10, "Value"="") -> ()  [unwired: 1 in, 2 out]
  n333 = control-ref of="Trigger Mode"() -> (w2:refnum<vi>)
  n334 = property class="DigNum (strict)"(reference=w2, "Value"=0) -> ()  [unwired: 1 in, 2 out]
  n335 = local write "Camera Status"(FALSE ("Camera Status")) -> ()
  n336 = property on="Scan Width" class="DigNum (strict)"("DisabledEnum"=w13) -> ()  [unwired: 2 in, 2 out]
  n337 = property on="Scan Line Delay" class="DigNum (strict)"("DisabledEnum"=w13) -> ()  [unwired: 2 in, 2 out]
  n338 = control-ref of="Scan Line Delay"() -> (w16:refnum<vi>)
  n339 = control-ref of="Scan Width"() -> (w19:refnum<vi>)
  n340 = control-ref of="Scan Line Time"() -> (w15:refnum<vi>)
  n341 = control-ref of="Scan Direction"() -> (w22:refnum<vi>)
  n342 = control-ref of="Scan Mode"() -> (w25:refnum<vi>)
  n343 = property class="CmbBox"(reference=w25, "Value"="", "Strings[]"=string[] [] ("Strings []")) -> ()  [unwired: 1 in, 2 out]
  n344 = property class="CmbBox"(reference=w22, "Strings[]"=string[] [] ("Strings []"), "Value"="") -> ()  [unwired: 1 in, 2 out]
  n345 = property class="DigNum (strict)"(reference=w16, "Value"=0.0) -> ()  [unwired: 1 in, 2 out]
  n346 = property class="DigNum (strict)"(reference=w19, "Value"=0.0) -> ()  [unwired: 1 in, 2 out]
  n347 = property class="DigNum (strict)"(reference=w15, "Value"=0.0) -> ()  [unwired: 1 in, 2 out]
  n348 = local write "Scan Direction Reset"(FALSE ("Boolean")) -> ()
  "Boolean" <- FALSE ("Boolean")
